vi "ParseVersionString.vi"(11 "VersionString":string) -> (0 "error out":errorcluster, 3 "Build spec version":T1)   [LabVIEW 2020, in "CICD.lvlib"]
doc: "Parse app version string according to the AbCellera convention. E.g. v0.4.0-rc2_htr404testing"
uses:
  CICD.lvlib
  <vilib>/AppBuilder/AB_API_Simple/Build Specification Version.ctl
  <vilib>/AppBuilder/AB_API_Simple/NI_App_Builder_API.lvlib
  <vilib>/regexp/Match Regular Expression.xnode
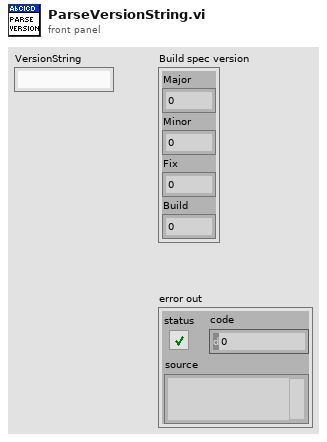
[diagram p1: front panel]
types:
  T1 = typedef "NI_App_Builder_API.lvlib/Build Specification Version.ctl" = cluster{"Major":u16, "Minor":u16, "Fix":u16, "Build":u16}
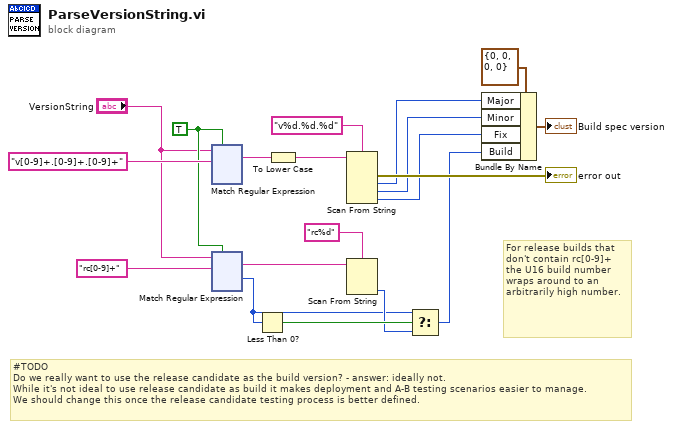
[diagram p0: block diagram]
diagram:
  w9 = TRUE ("ignore case? (F)")
  # "For release builds that don't contain rc[0-9]+ the U16 build number wraps around to an arbitrarily high number."
  # "#TODO\nDo we really want to use the release candidate as the build version? - answer: ideally not.\nWhile it's not ideal to use release candidate as build it makes deployment and A-B testing scenarios easier to manage.\nWe should change this once the release candidate testing process is better defined."
  n1 = xnode "Match Regular Expression"("input string"="VersionString", "regular expression"="v[0-9]+.[0-9]+.[0-9]+", "ignore case? (F)"=w9) -> ("whole match"=w7:string)  [unwired: 3 in, 4 out]
  n2 = xnode "Match Regular Expression"("input string"="VersionString", "regular expression"="rc[0-9]+", "ignore case? (F)"=w9) -> ("whole match"=w5:string, "offset past match"=w1:i32)  [unwired: 3 in, 3 out]
  n3 = Less Than 0?(x=w1) -> (x < 0?=w4:bool)
  n4 = To Lower Case(string=w7) -> (all lower case string=w17:string)
  n5 = Scan From String(format string="v%d.%d.%d", input string=w17) -> (error out=→"error out":errorcluster, output 1=w15:i32, output 2=w14:i32, output 3=w13:i32)  [unwired: 5 in, 2 out]
  n6 = Scan From String(format string="rc%d", input string=w5) -> (output 1=w2:i32)  [unwired: 3 in, 3 out]
  n7 = Select(t=w1, s=w4, f=w2) -> (s? t:f=w3:i32)
  n8 = Bundle By Name(cluster=T1 {"Major"=0, "Minor"=0, "Fix"=0, "Build"=0} ("Build Specification Version"), "Major"=w15, "Minor"=w14, "Fix"=w13, "Build"=w3) -> (→"Build spec version":T1)
